vi "_ValidateComment.vi"(4 "Expt#":i32, 7 "Comment":string) -> (0 "Error":string, 1 "ParamValue":dbl, 2 "SourceType":string, 3 "Valid":bool)   [LabVIEW 2012]
uses:
  <vilib>/regexp/Match Regular Expression.xnode
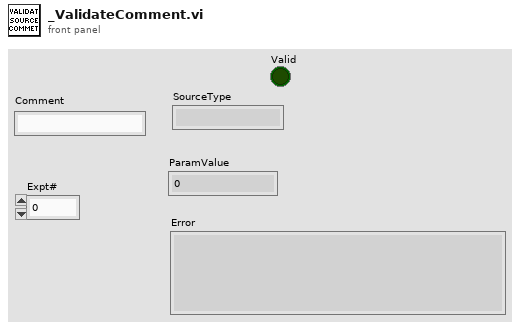
[diagram p1: front panel]
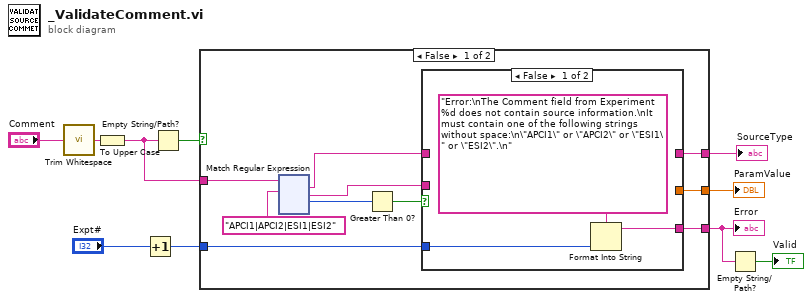
[diagram p0: block diagram]
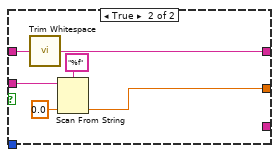
[diagram p2: hidden frame]
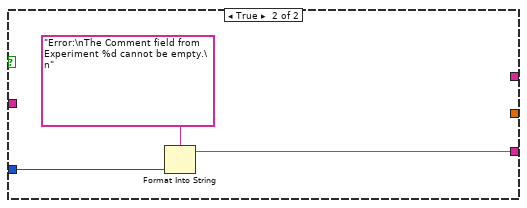
[diagram p3: hidden frame]
diagram:
  n1 = call <vilib>:"Trim Whitespace.vi"("string"="Comment") -> ("trimmed string"=w7:string)  [unwired: 1 in]
  n2 = To Upper Case(1:w7) -> (0:w6:string)
  n3 = Increment(x="Expt#") -> (x+1=w1:i32)
  n4 = Empty String/Path?(string/path=w6) -> (empty?=w9:bool)
  n5 = case shown="False" w9 {
    tunnel: w1 -> [w16 w142]
    tunnel: [w15 w141] -> w3
    tunnel: w6 -> [w19 _]
    tunnel: [w12 _] -> w5
    tunnel: [w11 _] -> w4
    frame False {
      n6 = xnode "Match Regular Expression"("input string"=w19, "regular expression"="APCI1|APCI2|ESI1|ESI2") -> ("whole match"=w14:string, "after match"=w13:string, "offset past match"=w18:i32)  [unwired: 4 in, 2 out]
      n7 = Greater Than 0?(x=w18) -> (x > 0?=w17:bool)
      n8 = case shown="False" w17 {
        tunnel: w16 -> [w22 _]
        tunnel: [w21 _] -> w15
        tunnel: w14 -> [_ w29]
        tunnel: w13 -> [_ w28]
        tunnel: [_ w25] -> w12
        tunnel: [_ w24] -> w11
        frame False {
          n9 = Format Into String(format string="Error:\nThe Comment field from Experiment %d does not contain source information.\nIt must contain one of the following strings without space:\n\"APCI1\" or \"APCI2\" or \"ESI1\" or \"ESI2\".\n", w22) -> (resulting string=w21:string)  [unwired: 2 in, 1 out]
        }
        frame True {
          n10 = call <vilib>:"Trim Whitespace.vi"("string"=w29) -> ("trimmed string"=w25:string)  [unwired: 1 in]
          n11 = Scan From String(format string="%f", input string=w28, default 1=0.0 ("default value 1")) -> (output 1=w24:dbl)  [unwired: 2 in, 3 out]
        }
      }
    }
    frame True {
      n12 = Format Into String(format string="Error:\nThe Comment field from Experiment %d cannot be empty.\n", w142) -> (resulting string=w141:string)  [unwired: 2 in, 1 out]
    }
  }
  "Error" <- w3
  "SourceType" <- w5
  "ParamValue" <- w4
  n13 = Empty String/Path?(string/path=w3) -> (empty?=→"Valid":bool)
